vi "WILT.vi"() -> ()   [LabVIEW 2016] (continued)
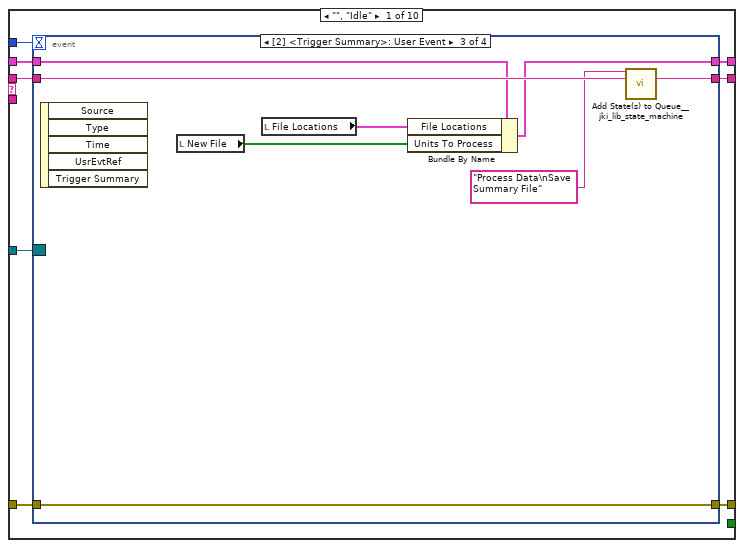
[diagram p2: hidden frame]
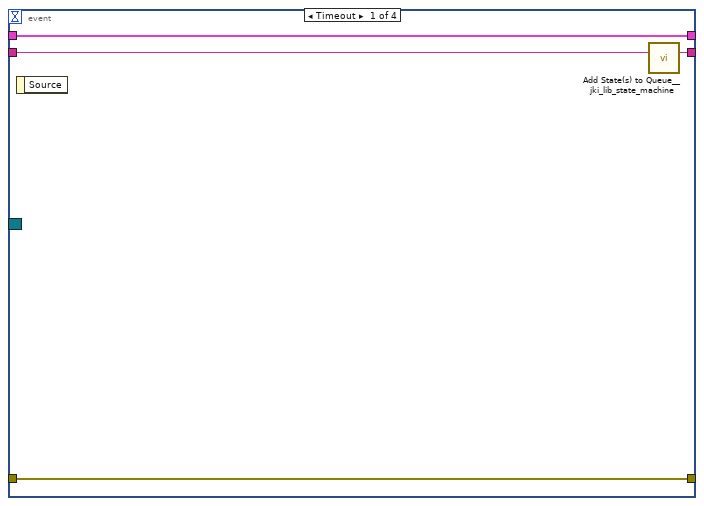
[diagram p3: hidden frame]
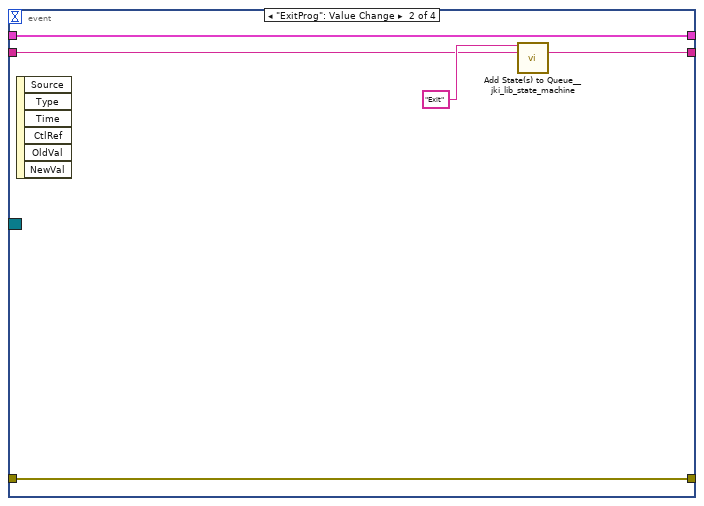
[diagram p4: hidden frame]
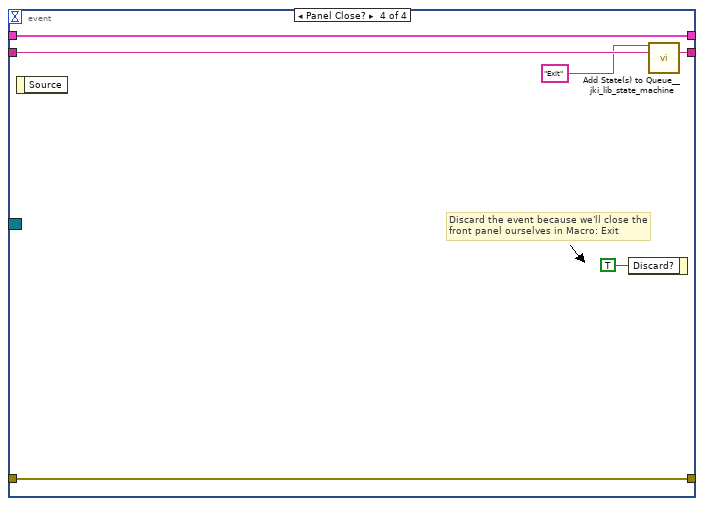
[diagram p5: hidden frame]
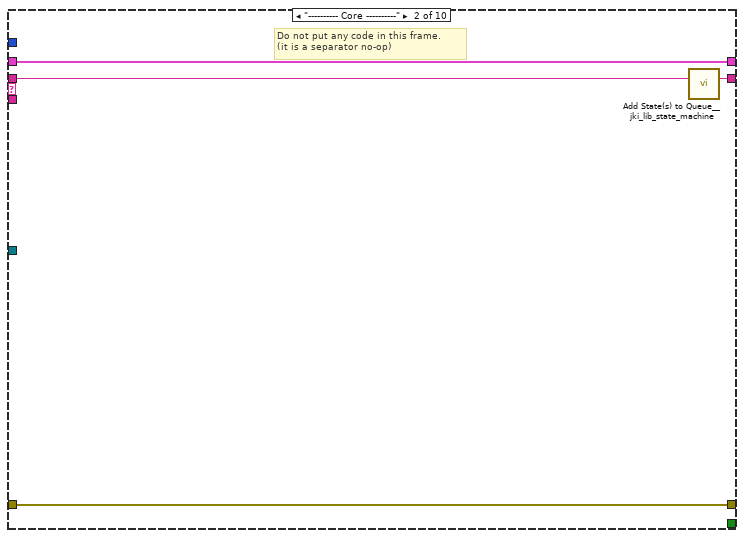
[diagram p6: hidden frame]
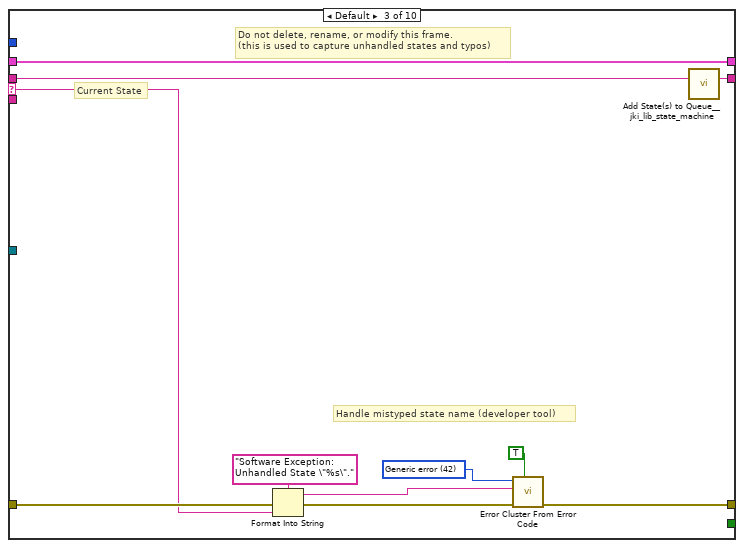
[diagram p7: hidden frame]
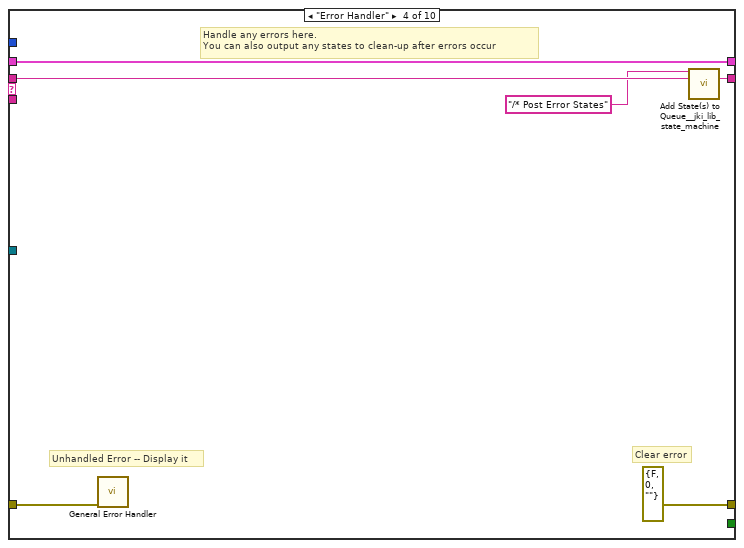
[diagram p8: hidden frame]
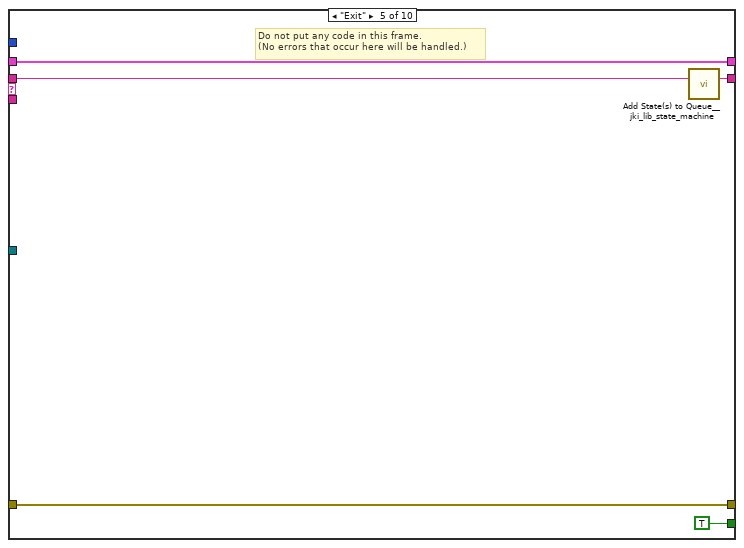
[diagram p9: hidden frame]
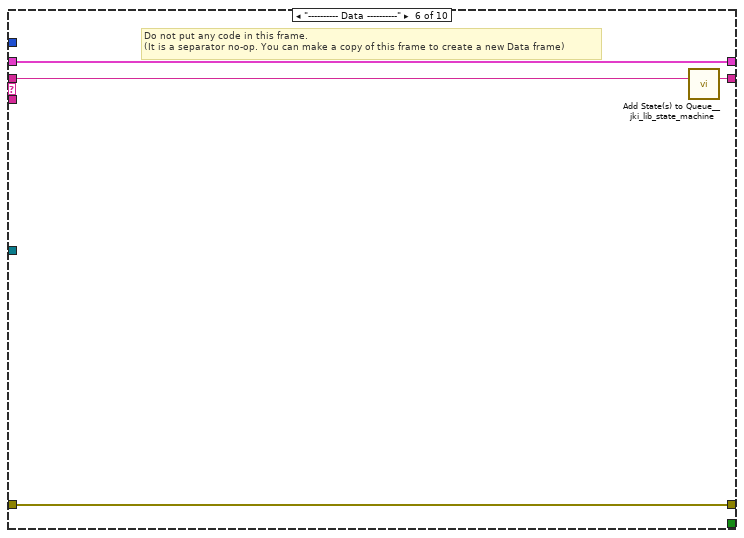
[diagram p10: hidden frame]
        n2035 = call <vilib>:"Add State(s) to Queue__jki_lib_state_machine.vi"("State(s) in (\"\")"=w4584) -> ("States Out"=w4583:string)  [unwired: 14 in]
      }
      frame "Update Filenames" {
        # "This takes alot of time to do...i cannot have 1 sec scan rate\nat this time...I set to 10 sec"
        n2036 = Unbundle By Name(w4604) -> ("First Time Through?"=w4601:bool[], "File Refnums"=w4587:refnum<file>[])
        n2037 = local read "Station Test State Cluster 2"() -> (w4586:T7)
        n2038 = local read "File Locations"() -> (w4602:T17[])
        n2039 = Wait on Notification(notifier=w4592, error in (no error)=w4591) -> (notification=w4589:T3[], error out=w4590:errorcluster)  [unwired: 2 in, 2 out]
        n2040 = call "WILT Save File.vi"("File Locations"=w4602, "Station Test State Cluster 2"=w4586, "Array in"=w4589, "File References In"=w4587, "Fisrt Time Through?"=w4601, "Error In"=w4590) -> ("File Locations Out"=w4600:T17[], "First Time Through Out"=w4585:bool[], "File References Out"=w4588:refnum<file>[], "New File"=w4599:bool[], "Error Out"=w4595:errorcluster)  [unwired: 5 in]
        "New File" <- w4599
        n2041 = Or Array Elements(Boolean array=w4599) -> (logical OR=w4598:bool)
        n2042 = case shown="True" w4598 {
          tunnel: w4597 -> [w4609 w4614]
          tunnel: [w4609 w4613] -> w4596
          tunnel: w4595 -> [w4608 w4612]
          tunnel: [w4608 w4611] -> w4594
          tunnel: ["" "Prepare for Save"] -> w4593
          frame False {
          }
          frame True {
            n2043 = Generate User Event(user event=w4614, event data cluster=TRUE ("Trigger"), error in=w4612) -> (user event out=w4613:refnum<user-event>, error out=w4611:errorcluster)  [unwired: 1 in]
          }
        }
        n2044 = Bundle By Name(cluster=w4604, "File Locations"=w4600, "First Time Through?"=w4585, "File Refnums"=w4588) -> (w4603:T36)
        n2045 = call <vilib>:"Add State(s) to Queue__jki_lib_state_machine.vi"("State(s) in Front (\"\")"=w4593, "State(s) in (\"\")"=w4606) -> ("States Out"=w4605:string)  [unwired: 13 in]
      }
    }
    n2046 = local read "Debug 2"() -> (w4468:bool)
    n2047 = case shown="False" w4468 {
      tunnel: w4471 -> [_ w4486]
      tunnel: [w4481 w4483] -> w4469
      tunnel: w4470 -> [w4481 w4485]
      frame False {
      }
      frame True {
        n2048 = Build Array (concatenate)(w4485, w4486) -> (w4482:string[])
        "Test State array 4" <- w4482
        n2049 = Array Size(array=w4482) -> (size(s)=w4484:i32)
        n2050 = case shown="100" w4484 {
          tunnel: [w4487 w4490] -> w4483
          tunnel: w4482 -> [w4487 w4491]
          frame 0, Default {
          }
          frame 100 {
            n2051 = Delete From Array(array=w4491, length=5, index=0) -> (array with subset deleted=w4490:string[])  [unwired: 1 out]
          }
        }
      }
    }
  }
  n2052 = while "Summary File Processing" {
    shift-right: [w4620] -> _
    shift-left: _ -> [w4619]
    shift-right: [w4623] -> _
    shift-left: _ -> [w4617]
    shift-right: [w4622] -> _
    shift-left: w48 -> [w4624]
    tunnel: w43 -> [w4616]
    stop <- w4621 stop-if-true
    w4618 = -1  # Timeout
    # "Summary File Processing"
    n2053 = call <vilib>:"Parse State Queue__jki_lib_state_machine.vi"("State Queue"=w4624, "Error In (no error)"=w4617) -> ("Remaining States"=w4626:string, "Current State"=w4627:string, "Arguments"=w4625:string)  [unwired: 11 in]
    n2054 = case shown="\"Process Data\"" w4627 {
      selector: w4627 -> [_ _ w4663 _ _ _ _ _ _ _]
      tunnel: w4626 -> [w4635 w4662 w4667 w4679 w4684 w4688 w4695 w4704 w4715 w4723]
      tunnel: w4625 -> [_ _ _ _ _ _ _ _ _ _]
      tunnel: w4619 -> [w4633 w4659 w4665 w4676 w4682 w4685 _ w4701 w4710 w4721]
      tunnel: [w4632 w4660 w4669 errorcluster {"status"=FALSE, "code"=0, "source"=""} ("error out") w4681 w4686 w4692 w4702 w4713 w4716] -> w4623
      tunnel: w4617 -> [w4631 w4660 w4668 w4675 w4681 w4686 w4692 w4702 w4713 w4717]
      tunnel: [w4634 w4661 w4666 w4678 w4683 w4687 w4694 w4703 w4714 w4722] -> w4622
      tunnel: [_ _ _ _ TRUE _ _ _ _ _] -> w4621
      tunnel: [w4630 w4659 w4665 w4676 w4682 w4685 w4693 w4701 w4709 w4721] -> w4620
      tunnel: w4618 -> [w4629 _ _ _ _ _ _ _ _ _]
      tunnel: w4616 -> [w4628 _ _ _ _ _ _ _ _ _]
      frame "", "Idle" {
        n2055 = event shown="[2] <Trigger Summary>: User Event" {
          selector: w4628 -> [_ _ _ _]
          dyn-events: _ -> [_ _ _ _]
          timeout: w4629 -> [_ _ _ _]
          tunnel: w4635 -> [w4639 w4641 w4651 w4658]
          tunnel: [w4638 w4642 w4652 w4657] -> w4634
          tunnel: w4633 -> [w4636 w4644 w4650 w4655]
          tunnel: [w4637 w4640 w4645 w4656] -> w4632
          tunnel: w4631 -> [w4637 w4640 w4645 w4656]
          tunnel: [w4636 w4644 w4649 w4655] -> w4630
          event Timeout {
            n2056 = event-data() -> ()  [unwired: 1 in, 1 out]
            n2057 = call <vilib>:"Add State(s) to Queue__jki_lib_state_machine.vi"("State(s) in (\"\")"=w4639) -> ("States Out"=w4638:string)  [unwired: 14 in]
          }
          event "ExitProg": Value Change {
            n2058 = event-data() -> ()  [unwired: 1 in, 6 out]
            n2059 = call <vilib>:"Add State(s) to Queue__jki_lib_state_machine.vi"("State(s) in Front (\"\")"="Exit" ("State(s) in Front (\"\")"), "State(s) in (\"\")"=w4641) -> ("States Out"=w4642:string)  [unwired: 13 in]
          }
          event User Event {
            n2060 = event-data() -> ()  [unwired: 1 in, 5 out]
            n2061 = local read "New File"() -> (w4648:bool[])
            n2062 = local read "File Locations"() -> (w4646:T17[])
            n2063 = Bundle By Name(cluster=w4650, "File Locations"=w4646, "Units To Process"=w4648) -> (w4649:T37)
            n2064 = call <vilib>:"Add State(s) to Queue__jki_lib_state_machine.vi"("State(s) in Front (\"\")"="Process Data\nSave Summary File" ("State(s) in Front (\"\")"), "State(s) in (\"\")"=w4651) -> ("States Out"=w4652:string)  [unwired: 13 in]
          }
          event Panel Close? {
            # "Discard the event because we'll close the front panel ourselves in Macro: Exit"
            n2065 = event-data() -> ()  [unwired: 1 in, 1 out]
            n2066 = event-data("Discard?"=TRUE) -> ()  [unwired: 1 in, 1 out]
            n2067 = call <vilib>:"Add State(s) to Queue__jki_lib_state_machine.vi"("State(s) in Front (\"\")"="Exit", "State(s) in (\"\")"=w4658) -> ("States Out"=w4657:string)  [unwired: 13 in]
          }
        }
      }
      frame "---------- Core ----------" {
        # "Do not put any code in this frame.\n(it is a separator no-op)"
        n2068 = call <vilib>:"Add State(s) to Queue__jki_lib_state_machine.vi"("State(s) in (\"\")"=w4662) -> ("States Out"=w4661:string)  [unwired: 14 in]
      }
      frame Default {
        w4672 = 42 items=["No error", "Argument error", "Memory is full", "Out of zone", "End of file", "File already open", "Generic file I/O error", "File not found", "File permission error", "Disk is full", "Duplicate path", "Too many files open", "System feature not enabled", "Resource file not found", "Cannot add resource", "Resource not found", "Image not found", "Image memory error", "Pen does not exist", "Config type invalid", "Config token not found", "Config parse error", "Config memory error", "Bad external code format", "Bad external code offset", "External code not present", "Null window", "Destroy window error", "Null menu", "Print aborted", "Bad print record", "Print driver error", "Windows error during printing", "Memory error during printing", "Print dialog error", "Generic print error", "Invalid device refnum", "Device not found", "Device parameter error", "Device unit error", "Cannot open device", "Device call aborted", "Generic error", "Cancelled by user", "Object ID too low", "Object ID too high", "Object not in heap", "Unknown heap", "Unknown object (invalid DefProc)", "Unknown object (DefProc not in table)", "Message out of range", "Invalid (null) method", "Unknown message", "Manager call not supported", "Bad address", "Network operation in progress", "Network operation timed out", "Connection is busy", "Network attribute not supported", "Network error", "Address in use", "System out of memory", "Connection aborted", "Connection refused", "Not connected", "Already connected", "Connection closed", "Initialization error (interapplication manager)", "Bad occurrence", "Wait on unbound occurrence handler", "Occurrence queue overflow", "Datalog type conflict", "Unused", "Unrecognized type (interapplication manager)", "Memory corrupt", "Failed to make temporary DLL", "Old CIN version", "Drag socket not found", "Failed to load drop-object", "Failed to register OLE object", "Failed to release OLE object", "Format specifier type mismatch", "Unknown format specifier", "Too few format specifiers", "Too many format specifiers", "Scan failed", "Newer CIN version", "Error converting to variant", "Runtime menu error", "Password tampered", "Variant attribute not found", "Incompatible variant data type", "Event data is not available", "Event Store is not present", "Occurrence is not found", "Event Queue is not created", "Event info is not available", "Refnum passed is NULL", "Error retrieving Class GUID", "Error retrieving CoClass GUID", "Error retrieving TypeLib GUID.", "Bad built application magic bytes.", "Specific driver is different from the specific driver associated with the Logical Name.", "There is no session opened to the class driver.", "Max Error", "MAX - Error with config objects", "MAX - Error loading configuration", "MAX - Group not supported"]
        # "Current State"
        # "Do not delete, rename, or modify this frame.\n(this is used to capture unhandled states and typos)"
        # "Handle mistyped state name (developer tool)"
        n2069 = Format Into String(format string="Software Exception: Unhandled State \"%s\"." ("message"), error in=w4668, w4663) -> (resulting string=w4671:string, error out=w4670:errorcluster)  [unwired: 1 in]
        n2070 = call <vilib>:"Error Cluster From Error Code.vi"("show call chain? (False)"=TRUE, "error in (no error)"=w4670, "error message (\"\")"=w4671, "error code (0)"=w4672) -> ("error out"=w4669:errorcluster)  [unwired: 5 in]
        n2071 = call <vilib>:"Add State(s) to Queue__jki_lib_state_machine.vi"("State(s) in (\"\")"=w4667) -> ("States Out"=w4666:string)  [unwired: 14 in]
      }
      frame "Error Handler" {
        # "Unhandled Error -- Display it"
        # "Handle any errors here.\nYou can also output any states to clean-up after errors occur"
        # "Clear error"
        n2072 = call <vilib>:"General Error Handler.vi"("error in (no error)"=w4675) -> ()  [unwired: 10 in, 5 out]
        n2073 = call <vilib>:"Add State(s) to Queue__jki_lib_state_machine.vi"("State(s) in Front (\"\")"="/* Post Error States", "State(s) in (\"\")"=w4679) -> ("States Out"=w4678:string)  [unwired: 13 in]
      }
      frame "Exit" {
        # "Do not put any code in this frame.\n(No errors that occur here will be handled.)"
        n2074 = call <vilib>:"Add State(s) to Queue__jki_lib_state_machine.vi"("State(s) in (\"\")"=w4684) -> ("States Out"=w4683:string)  [unwired: 14 in]
      }
      frame "---------- Data ----------" {
        # "Do not put any code in this frame.\n(It is a separator no-op. You can make a copy of this frame to create a new Data frame)"
        n2075 = call <vilib>:"Add State(s) to Queue__jki_lib_state_machine.vi"("State(s) in (\"\")"=w4688) -> ("States Out"=w4687:string)  [unwired: 14 in]
      }
      frame "Data: Initialize" {
        n2076 = while {
          tunnel: [w4698] -> w4691
          tunnel: [w4696] -> w4690
          tunnel: [w4697] -> w4689
          stop <- w4700 stop-if-true
          w4696 = T9[] [{"Cycle Time (Minutes)"=0.0, "L1 Current (Amps)"=0.0, "L2 Current (Amps)"=0.0, "TC Temperature (Deg F)"=0.0, "Voltage (Volts)"=0.0, "Voltage-208 (Volts)"=0.0, "208V Switch (Ohms)"=0.0, "Cycle Number"=0}, {"Cycle Time (Minutes)"=0.0, "L1 Current (Amps)"=0.0, "L2 Current (Amps)"=0.0, "TC Temperature (Deg F)"=0.0, "Voltage (Volts)"=0.0, "Voltage-208 (Volts)"=0.0, "208V Switch (Ohms)"=0.0, "Cycle Number"=0}, {"Cycle Time (Minutes)"=0.0, "L1 Current (Amps)"=0.0, "L2 Current (Amps)"=0.0, "TC Temperature (Deg F)"=0.0, "Voltage (Volts)"=0.0, "Voltage-208 (Volts)"=0.0, "208V Switch (Ohms)"=0.0, "Cycle Number"=0}, {"Cycle Time (Minutes)"=0.0, "L1 Current (Amps)"=0.0, "L2 Current (Amps)"=0.0, "TC Temperature (Deg F)"=0.0, "Voltage (Volts)"=0.0, "Voltage-208 (Volts)"=0.0, "208V Switch (Ohms)"=0.0, "Cycle Number"=0}, {"Cycle Time (Minutes)"=0.0, "L1 Current (Amps)"=0.0, "L2 Current (Amps)"=0.0, "TC Temperature (Deg F)"=0.0, "Voltage (Volts)"=0.0, "Voltage-208 (Volts)"=0.0, "208V Switch (Ohms)"=0.0, "Cycle Number"=0}, {"Cycle Time (Minutes)"=0.0, "L1 Current (Amps)"=0.0, "L2 Current (Amps)"=0.0, "TC Temperature (Deg F)"=0.0, "Voltage (Volts)"=0.0, "Voltage-208 (Volts)"=0.0, "208V Switch (Ohms)"=0.0, "Cycle Number"=0}, {"Cycle Time (Minutes)"=0.0, "L1 Current (Amps)"=0.0, "L2 Current (Amps)"=0.0, "TC Temperature (Deg F)"=0.0, "Voltage (Volts)"=0.0, "Voltage-208 (Volts)"=0.0, "208V Switch (Ohms)"=0.0, "Cycle Number"=0}, {"Cycle Time (Minutes)"=0.0, "L1 Current (Amps)"=0.0, "L2 Current (Amps)"=0.0, "TC Temperature (Deg F)"=0.0, "Voltage (Volts)"=0.0, "Voltage-208 (Volts)"=0.0, "208V Switch (Ohms)"=0.0, "Cycle Number"=0}, {"Cycle Time (Minutes)"=0.0, "L1 Current (Amps)"=0.0, "L2 Current (Amps)"=0.0, "TC Temperature (Deg F)"=0.0, "Voltage (Volts)"=0.0, "Voltage-208 (Volts)"=0.0, "208V Switch (Ohms)"=0.0, "Cycle Number"=0}, {"Cycle Time (Minutes)"=0.0, "L1 Current (Amps)"=0.0, "L2 Current (Amps)"=0.0, "TC Temperature (Deg F)"=0.0, "Voltage (Volts)"=0.0, "Voltage-208 (Volts)"=0.0, "208V Switch (Ohms)"=0.0, "Cycle Number"=0}, {"Cycle Time (Minutes)"=0.0, "L1 Current (Amps)"=0.0, "L2 Current (Amps)"=0.0, "TC Temperature (Deg F)"=0.0, "Voltage (Volts)"=0.0, "Voltage-208 (Volts)"=0.0, "208V Switch (Ohms)"=0.0, "Cycle Number"=0}, {"Cycle Time (Minutes)"=0.0, "L1 Current (Amps)"=0.0, "L2 Current (Amps)"=0.0, "TC Temperature (Deg F)"=0.0, "Voltage (Volts)"=0.0, "Voltage-208 (Volts)"=0.0, "208V Switch (Ohms)"=0.0, "Cycle Number"=0}, {"Cycle Time (Minutes)"=0.0, "L1 Current (Amps)"=0.0, "L2 Current (Amps)"=0.0, "TC Temperature (Deg F)"=0.0, "Voltage (Volts)"=0.0, "Voltage-208 (Volts)"=0.0, "208V Switch (Ohms)"=0.0, "Cycle Number"=0}, {"Cycle Time (Minutes)"=0.0, "L1 Current (Amps)"=0.0, "L2 Current (Amps)"=0.0, "TC Temperature (Deg F)"=0.0, "Voltage (Volts)"=0.0, "Voltage-208 (Volts)"=0.0, "208V Switch (Ohms)"=0.0, "Cycle Number"=0}, {"Cycle Time (Minutes)"=0.0, "L1 Current (Amps)"=0.0, "L2 Current (Amps)"=0.0, "TC Temperature (Deg F)"=0.0, "Voltage (Volts)"=0.0, "Voltage-208 (Volts)"=0.0, "208V Switch (Ohms)"=0.0, "Cycle Number"=0}, {"Cycle Time (Minutes)"=0.0, "L1 Current (Amps)"=0.0, "L2 Current (Amps)"=0.0, "TC Temperature (Deg F)"=0.0, "Voltage (Volts)"=0.0, "Voltage-208 (Volts)"=0.0, "208V Switch (Ohms)"=0.0, "Cycle Number"=0}, {"Cycle Time (Minutes)"=0.0, "L1 Current (Amps)"=0.0, "L2 Current (Amps)"=0.0, "TC Temperature (Deg F)"=0.0, "Voltage (Volts)"=0.0, "Voltage-208 (Volts)"=0.0, "208V Switch (Ohms)"=0.0, "Cycle Number"=0}, {"Cycle Time (Minutes)"=0.0, "L1 Current (Amps)"=0.0, "L2 Current (Amps)"=0.0, "TC Temperature (Deg F)"=0.0, "Voltage (Volts)"=0.0, "Voltage-208 (Volts)"=0.0, "208V Switch (Ohms)"=0.0, "Cycle Number"=0}, {"Cycle Time (Minutes)"=0.0, "L1 Current (Amps)"=0.0, "L2 Current (Amps)"=0.0, "TC Temperature (Deg F)"=0.0, "Voltage (Volts)"=0.0, "Voltage-208 (Volts)"=0.0, "208V Switch (Ohms)"=0.0, "Cycle Number"=0}, {"Cycle Time (Minutes)"=0.0, "L1 Current (Amps)"=0.0, "L2 Current (Amps)"=0.0, "TC Temperature (Deg F)"=0.0, "Voltage (Volts)"=0.0, "Voltage-208 (Volts)"=0.0, "208V Switch (Ohms)"=0.0, "Cycle Number"=0}, {"Cycle Time (Minutes)"=0.0, "L1 Current (Amps)"=0.0, "L2 Current (Amps)"=0.0, "TC Temperature (Deg F)"=0.0, "Voltage (Volts)"=0.0, "Voltage-208 (Volts)"=0.0, "208V Switch (Ohms)"=0.0, "Cycle Number"=0}, {"Cycle Time (Minutes)"=0.0, "L1 Current (Amps)"=0.0, "L2 Current (Amps)"=0.0, "TC Temperature (Deg F)"=0.0, "Voltage (Volts)"=0.0, "Voltage-208 (Volts)"=0.0, "208V Switch (Ohms)"=0.0, "Cycle Number"=0}, {"Cycle Time (Minutes)"=0.0, "L1 Current (Amps)"=0.0, "L2 Current (Amps)"=0.0, "TC Temperature (Deg F)"=0.0, "Voltage (Volts)"=0.0, "Voltage-208 (Volts)"=0.0, "208V Switch (Ohms)"=0.0, "Cycle Number"=0}, {"Cycle Time (Minutes)"=0.0, "L1 Current (Amps)"=0.0, "L2 Current (Amps)"=0.0, "TC Temperature (Deg F)"=0.0, "Voltage (Volts)"=0.0, "Voltage-208 (Volts)"=0.0, "208V Switch (Ohms)"=0.0, "Cycle Number"=0}, {"Cycle Time (Minutes)"=0.0, "L1 Current (Amps)"=0.0, "L2 Current (Amps)"=0.0, "TC Temperature (Deg F)"=0.0, "Voltage (Volts)"=0.0, "Voltage-208 (Volts)"=0.0, "208V Switch (Ohms)"=0.0, "Cycle Number"=0}, {"Cycle Time (Minutes)"=0.0, "L1 Current (Amps)"=0.0, "L2 Current (Amps)"=0.0, "TC Temperature (Deg F)"=0.0, "Voltage (Volts)"=0.0, "Voltage-208 (Volts)"=0.0, "208V Switch (Ohms)"=0.0, "Cycle Number"=0}, {"Cycle Time (Minutes)"=0.0, "L1 Current (Amps)"=0.0, "L2 Current (Amps)"=0.0, "TC Temperature (Deg F)"=0.0, "Voltage (Volts)"=0.0, "Voltage-208 (Volts)"=0.0, "208V Switch (Ohms)"=0.0, "Cycle Number"=0}, {"Cycle Time (Minutes)"=0.0, "L1 Current (Amps)"=0.0, "L2 Current (Amps)"=0.0, "TC Temperature (Deg F)"=0.0, "Voltage (Volts)"=0.0, "Voltage-208 (Volts)"=0.0, "208V Switch (Ohms)"=0.0, "Cycle Number"=0}, {"Cycle Time (Minutes)"=0.0, "L1 Current (Amps)"=0.0, "L2 Current (Amps)"=0.0, "TC Temperature (Deg F)"=0.0, "Voltage (Volts)"=0.0, "Voltage-208 (Volts)"=0.0, "208V Switch (Ohms)"=0.0, "Cycle Number"=0}, {"Cycle Time (Minutes)"=0.0, "L1 Current (Amps)"=0.0, "L2 Current (Amps)"=0.0, "TC Temperature (Deg F)"=0.0, "Voltage (Volts)"=0.0, "Voltage-208 (Volts)"=0.0, "208V Switch (Ohms)"=0.0, "Cycle Number"=0}, {"Cycle Time (Minutes)"=0.0, "L1 Current (Amps)"=0.0, "L2 Current (Amps)"=0.0, "TC Temperature (Deg F)"=0.0, "Voltage (Volts)"=0.0, "Voltage-208 (Volts)"=0.0, "208V Switch (Ohms)"=0.0, "Cycle Number"=0}, {"Cycle Time (Minutes)"=0.0, "L1 Current (Amps)"=0.0, "L2 Current (Amps)"=0.0, "TC Temperature (Deg F)"=0.0, "Voltage (Volts)"=0.0, "Voltage-208 (Volts)"=0.0, "208V Switch (Ohms)"=0.0, "Cycle Number"=0}, {"Cycle Time (Minutes)"=0.0, "L1 Current (Amps)"=0.0, "L2 Current (Amps)"=0.0, "TC Temperature (Deg F)"=0.0, "Voltage (Volts)"=0.0, "Voltage-208 (Volts)"=0.0, "208V Switch (Ohms)"=0.0, "Cycle Number"=0}, {"Cycle Time (Minutes)"=0.0, "L1 Current (Amps)"=0.0, "L2 Current (Amps)"=0.0, "TC Temperature (Deg F)"=0.0, "Voltage (Volts)"=0.0, "Voltage-208 (Volts)"=0.0, "208V Switch (Ohms)"=0.0, "Cycle Number"=0}, {"Cycle Time (Minutes)"=0.0, "L1 Current (Amps)"=0.0, "L2 Current (Amps)"=0.0, "TC Temperature (Deg F)"=0.0, "Voltage (Volts)"=0.0, "Voltage-208 (Volts)"=0.0, "208V Switch (Ohms)"=0.0, "Cycle Number"=0}, {"Cycle Time (Minutes)"=0.0, "L1 Current (Amps)"=0.0, "L2 Current (Amps)"=0.0, "TC Temperature (Deg F)"=0.0, "Voltage (Volts)"=0.0, "Voltage-208 (Volts)"=0.0, "208V Switch (Ohms)"=0.0, "Cycle Number"=0}, {"Cycle Time (Minutes)"=0.0, "L1 Current (Amps)"=0.0, "L2 Current (Amps)"=0.0, "TC Temperature (Deg F)"=0.0, "Voltage (Volts)"=0.0, "Voltage-208 (Volts)"=0.0, "208V Switch (Ohms)"=0.0, "Cycle Number"=0}, {"Cycle Time (Minutes)"=0.0, "L1 Current (Amps)"=0.0, "L2 Current (Amps)"=0.0, "TC Temperature (Deg F)"=0.0, "Voltage (Volts)"=0.0, "Voltage-208 (Volts)"=0.0, "208V Switch (Ohms)"=0.0, "Cycle Number"=0}, {"Cycle Time (Minutes)"=0.0, "L1 Current (Amps)"=0.0, "L2 Current (Amps)"=0.0, "TC Temperature (Deg F)"=0.0, "Voltage (Volts)"=0.0, "Voltage-208 (Volts)"=0.0, "208V Switch (Ohms)"=0.0, "Cycle Number"=0}, {"Cycle Time (Minutes)"=0.0, "L1 Current (Amps)"=0.0, "L2 Current (Amps)"=0.0, "TC Temperature (Deg F)"=0.0, "Voltage (Volts)"=0.0, "Voltage-208 (Volts)"=0.0, "208V Switch (Ohms)"=0.0, "Cycle Number"=0}, {"Cycle Time (Minutes)"=0.0, "L1 Current (Amps)"=0.0, "L2 Current (Amps)"=0.0, "TC Temperature (Deg F)"=0.0, "Voltage (Volts)"=0.0, "Voltage-208 (Volts)"=0.0, "208V Switch (Ohms)"=0.0, "Cycle Number"=0}, {"Cycle Time (Minutes)"=0.0, "L1 Current (Amps)"=0.0, "L2 Current (Amps)"=0.0, "TC Temperature (Deg F)"=0.0, "Voltage (Volts)"=0.0, "Voltage-208 (Volts)"=0.0, "208V Switch (Ohms)"=0.0, "Cycle Number"=0}, {"Cycle Time (Minutes)"=0.0, "L1 Current (Amps)"=0.0, "L2 Current (Amps)"=0.0, "TC Temperature (Deg F)"=0.0, "Voltage (Volts)"=0.0, "Voltage-208 (Volts)"=0.0, "208V Switch (Ohms)"=0.0, "Cycle Number"=0}, {"Cycle Time (Minutes)"=0.0, "L1 Current (Amps)"=0.0, "L2 Current (Amps)"=0.0, "TC Temperature (Deg F)"=0.0, "Voltage (Volts)"=0.0, "Voltage-208 (Volts)"=0.0, "208V Switch (Ohms)"=0.0, "Cycle Number"=0}, {"Cycle Time (Minutes)"=0.0, "L1 Current (Amps)"=0.0, "L2 Current (Amps)"=0.0, "TC Temperature (Deg F)"=0.0, "Voltage (Volts)"=0.0, "Voltage-208 (Volts)"=0.0, "208V Switch (Ohms)"=0.0, "Cycle Number"=0}, {"Cycle Time (Minutes)"=0.0, "L1 Current (Amps)"=0.0, "L2 Current (Amps)"=0.0, "TC Temperature (Deg F)"=0.0, "Voltage (Volts)"=0.0, "Voltage-208 (Volts)"=0.0, "208V Switch (Ohms)"=0.0, "Cycle Number"=0}, {"Cycle Time (Minutes)"=0.0, "L1 Current (Amps)"=0.0, "L2 Current (Amps)"=0.0, "TC Temperature (Deg F)"=0.0, "Voltage (Volts)"=0.0, "Voltage-208 (Volts)"=0.0, "208V Switch (Ohms)"=0.0, "Cycle Number"=0}, {"Cycle Time (Minutes)"=0.0, "L1 Current (Amps)"=0.0, "L2 Current (Amps)"=0.0, "TC Temperature (Deg F)"=0.0, "Voltage (Volts)"=0.0, "Voltage-208 (Volts)"=0.0, "208V Switch (Ohms)"=0.0, "Cycle Number"=0}, {"Cycle Time (Minutes)"=0.0, "L1 Current (Amps)"=0.0, "L2 Current (Amps)"=0.0, "TC Temperature (Deg F)"=0.0, "Voltage (Volts)"=0.0, "Voltage-208 (Volts)"=0.0, "208V Switch (Ohms)"=0.0, "Cycle Number"=0}, {"Cycle Time (Minutes)"=0.0, "L1 Current (Amps)"=0.0, "L2 Current (Amps)"=0.0, "TC Temperature (Deg F)"=0.0, "Voltage (Volts)"=0.0, "Voltage-208 (Volts)"=0.0, "208V Switch (Ohms)"=0.0, "Cycle Number"=0}, {"Cycle Time (Minutes)"=0.0, "L1 Current (Amps)"=0.0, "L2 Current (Amps)"=0.0, "TC Temperature (Deg F)"=0.0, "Voltage (Volts)"=0.0, "Voltage-208 (Volts)"=0.0, "208V Switch (Ohms)"=0.0, "Cycle Number"=0}, {"Cycle Time (Minutes)"=0.0, "L1 Current (Amps)"=0.0, "L2 Current (Amps)"=0.0, "TC Temperature (Deg F)"=0.0, "Voltage (Volts)"=0.0, "Voltage-208 (Volts)"=0.0, "208V Switch (Ohms)"=0.0, "Cycle Number"=0}, {"Cycle Time (Minutes)"=0.0, "L1 Current (Amps)"=0.0, "L2 Current (Amps)"=0.0, "TC Temperature (Deg F)"=0.0, "Voltage (Volts)"=0.0, "Voltage-208 (Volts)"=0.0, "208V Switch (Ohms)"=0.0, "Cycle Number"=0}, {"Cycle Time (Minutes)"=0.0, "L1 Current (Amps)"=0.0, "L2 Current (Amps)"=0.0, "TC Temperature (Deg F)"=0.0, "Voltage (Volts)"=0.0, "Voltage-208 (Volts)"=0.0, "208V Switch (Ohms)"=0.0, "Cycle Number"=0}, {"Cycle Time (Minutes)"=0.0, "L1 Current (Amps)"=0.0, "L2 Current (Amps)"=0.0, "TC Temperature (Deg F)"=0.0, "Voltage (Volts)"=0.0, "Voltage-208 (Volts)"=0.0, "208V Switch (Ohms)"=0.0, "Cycle Number"=0}, {"Cycle Time (Minutes)"=0.0, "L1 Current (Amps)"=0.0, "L2 Current (Amps)"=0.0, "TC Temperature (Deg F)"=0.0, "Voltage (Volts)"=0.0, "Voltage-208 (Volts)"=0.0, "208V Switch (Ohms)"=0.0, "Cycle Number"=0}]  # WILT Summary Array
          w4697 = bool[] [FALSE, FALSE, FALSE, FALSE, FALSE, FALSE, FALSE, FALSE, FALSE, FALSE, FALSE, FALSE, FALSE, FALSE, FALSE, FALSE, FALSE, FALSE, FALSE, FALSE, FALSE, FALSE, FALSE, FALSE, FALSE, FALSE, FALSE, FALSE, FALSE, FALSE, FALSE, FALSE, FALSE, FALSE, FALSE, FALSE, FALSE, FALSE, FALSE, FALSE, FALSE, FALSE, FALSE, FALSE, FALSE, FALSE, FALSE, FALSE, FALSE, FALSE, FALSE, FALSE, FALSE, FALSE, FALSE, FALSE]  # Units To Process
          n2077 = local read "Initialization Complete"() -> (w4700:bool)
          n2078 = local read "File Locations"() -> (w4698:T17[])
          n2079 = Wait Until Next ms Multiple(millisecond multiple=u32 100) -> ()  [unwired: 1 out]
        }
        n2080 = Bundle("File Locations"=w4691, "WILT Summary Array"=w4690, "Units To Process"=w4689) -> (w4693:T37)  [unwired: 1 in]
        n2081 = call <vilib>:"Add State(s) to Queue__jki_lib_state_machine.vi"("State(s) in (\"\")"=w4695) -> ("States Out"=w4694:string)  [unwired: 14 in]
      }
      frame "---------- Summary File Process ----------" {
        n2082 = call <vilib>:"Add State(s) to Queue__jki_lib_state_machine.vi"("State(s) in (\"\")"=w4704) -> ("States Out"=w4703:string)  [unwired: 14 in]
      }
      frame "Process Data" {
        # "Loops through all files and computes\ncomplete files. Including Cycle Time"
        n2083 = Unbundle By Name(w4710) -> ("WILT Summary Array"=w4706:T9[], "Units To Process"=w4708:bool[], "File Locations"=w4712:T17[])
        n2084 = call "WILT Process Cycle Data.vi"("WILT Summary Input"=w4706, "Inverter File Headers"=string[] ["Date", "Time (24 Hour Format)", "Cycle Time (Minutes)", "L1 Current (Amps)", "L2 Current (Amps)", "TC Temperature (Deg F)", "Voltage (Volts)", "Voltage-208 (Volts)", "208V Switch (Ohms)", "Cycle Number"], "File Locations"=w4712, "New File"=w4708) -> ("Units to Process"=w4707:bool[], "WILT Summary Output"=w4705:T9[])  [unwired: 6 in]
        "Previous Run Statistics" <- w4705
        n2085 = Bundle By Name(cluster=w4710, "WILT Summary Array"=w4705, "Units To Process"=w4707) -> (w4709:T37)
        n2086 = call <vilib>:"Add State(s) to Queue__jki_lib_state_machine.vi"("State(s) in (\"\")"=w4715) -> ("States Out"=w4714:string)  [unwired: 14 in]
      }
      frame "Save Summary File" {
        # "This could consume memory\nkeep a watch"
        # "Loops through files and saves data\nto summary file by cycle number"
        n2087 = Unbundle By Name(w4721) -> ("Units To Process"=w4720:bool[], "File Locations"=w4719:T17[], "WILT Summary Array"=w4718:T9[])
        n2088 = for {
          tunnel: w4720 -> [w4728] mode=indexing
          tunnel: w4719 -> [w4727] mode=indexing
          tunnel: w4718 -> [w4726] mode=indexing
          shift-right: [w4724] -> w4716
          shift-left: w4717 -> [w4725]
          n2089 = case shown="True" w4728 {
            tunnel: w4727 -> [_ w4738]
            tunnel: w4726 -> [_ w4733]
            tunnel: w4725 -> [w4729 w4732]
            tunnel: [w4729 w4732] -> w4724
            frame False {
            }
            frame True {
              n2090 = Unbundle By Name(w4738) -> ("Data File Paths.Summary"=w4737:path)
              n2091 = call "WILT Format Summary File.vi"("WILT Summary Cluster Input"=w4733) -> ("Summary Data"=w4730:string[])  [unwired: 10 in]
              n2092 = call "Save File Check and Fix Summary File.vi"("LV Program"=Save_File_DOE_LabView_Program."Dryer", "file path (dialog if empty)"=w4737) -> ("Summary Path"=w4734:path)  [unwired: 8 in, 1 out]
              n2093 = call-poly <vilib>:"Write Delimited Spreadsheet.vi"("file path (dialog if empty)"=w4734, "1D data"=w4730, "append to file? (new file:F)"=TRUE, "delimiter (\\t)"="," ("delimiter (\\t)")) -> ()  [unwired: 10 in, 2 out]
            }
          }
        }
        n2094 = call <vilib>:"Add State(s) to Queue__jki_lib_state_machine.vi"("State(s) in (\"\")"=w4723) -> ("States Out"=w4722:string)  [unwired: 14 in]
      }
    }
  }
  n2095 = while {
    shift-right: [w4753] -> _
    shift-left: _ -> [w4752]
    shift-right: [w4756] -> w16
    shift-left: w18 -> [w4750]
    shift-right: [w4755] -> _
    shift-left: w53 -> [w4757]
    tunnel: w7 -> [w4749]
    tunnel: w6 -> [w4748]
    tunnel: w5 -> [w4747]
    tunnel: w4 -> [w4746]
    tunnel: w3 -> [w4745]
    tunnel: [w4744] -> w17
    tunnel: [w4743] -> w14
    tunnel: [w4742] -> w12
    tunnel: [w4741] -> w10
    tunnel: [w4740] -> w8
    i -> [w4739]
    stop <- w4754 stop-if-true
    w4751 = -1  # Timeout
    # "UI State Machine"
    n2096 = call <vilib>:"Parse State Queue__jki_lib_state_machine.vi"("State Queue"=w4757, "Error In (no error)"=w4750) -> ("Remaining States"=w4759:string, "Current State"=w4760:string, "Arguments"=w4758:string)  [unwired: 11 in]
    n2097 = case shown="\"\", \"Idle\"" w4760 {
      selector: w4760 -> [_ _ w4973 _ _ _ _ _]
      tunnel: w4759 -> [w4777 w4967 w4977 w4994 w5004 w5013 w5024 w5037]
      tunnel: w4758 -> [_ _ _ _ _ _ _ _]
      tunnel: w4752 -> [w4775 w4964 w4975 w4991 w5002 w5010 _ w5034]
      tunnel: [w4774 w4965 w4979 errorcluster {"status"=FALSE, "code"=0, "source"=""} ("error out") w5001 w5011 w5021 w5035] -> w4756
      tunnel: w4750 -> [w4773 w4965 w4978 w4990 w5001 w5011 w5021 w5035]
      tunnel: [w4776 w4966 w4976 w4993 w5003 w5012 w5023 w5036] -> w4755
      tunnel: [_ _ _ _ TRUE _ _ _] -> w4754
      tunnel: [w4772 w4964 w4975 w4991 w5002 w5010 w5022 w5034] -> w4753
      tunnel: w4751 -> [w4771 _ _ _ _ _ _ _]
      tunnel: w4749 -> [w4770 w4963 w4972 w4988 w4999 w5009 w5018 w5033]
      tunnel: w4748 -> [w4769 w4962 w4971 w4987 w4998 w5008 w5017 w5032]
      tunnel: w4747 -> [w4768 w4961 w4970 w4986 w4997 w5007 w5016 w5031]
      tunnel: w4746 -> [w4767 w4960 w4969 w4985 w4996 w5006 w5015 w5030]
      tunnel: w4745 -> [w4766 w4959 w4968 w4984 w4995 w5005 w5014 w5029]
      tunnel: [w4765 w4963 w4972 w4988 w4999 w5009 w5018 w5033] -> w4744
      tunnel: [w4764 w4962 w4971 w4987 w4998 w5008 w5017 w5032] -> w4743
      tunnel: [w4763 w4961 w4970 w4986 w4997 w5007 w5016 w5031] -> w4742
      tunnel: [w4762 w4960 w4969 w4985 w4996 w5006 w5015 w5030] -> w4741
      tunnel: [w4761 w4959 w4968 w4984 w4995 w5005 w5014 w5029] -> w4740
      frame "", "Idle" {
        n2098 = event shown="[2] \"GUI Aisle 4.\": Value Change" {
          selector: _ -> [_ _ _ _ _ _ _ _]
          dyn-events: _ -> [_ _ _ _ _ _ _ _]
          timeout: w4771 -> [_ _ _ _ _ _ _ _]
          tunnel: w4777 -> [w4787 w4796 w4818 w4848 w4878 w4908 w4938 w4958]
          tunnel: [w4786 w4795 w4817 w4849 w4879 w4909 w4939 w4957] -> w4776
          tunnel: w4775 -> [w4784 w4794 w4819 w4847 w4877 w4907 w4937 w4955]
          tunnel: [w4785 w4793 w4812 w4841 w4871 w4898 w4933 w4956] -> w4774
          tunnel: w4773 -> [w4785 w4793 w4804 w4837 w4864 w4899 w4926 w4956]
          tunnel: [w4784 w4794 w4819 w4847 w4877 w4907 w4937 w4955] -> w4772
          tunnel: w4770 -> [w4782 w4792 w4810 w4840 w4870 w4893 w4930 w4952]
          tunnel: w4769 -> [w4781 w4791 w4809 w4839 w4869 w4892 w4928 w4951]
          tunnel: w4768 -> [w4780 w4790 w4808 w4838 w4868 w4890 w4920 w4950]
          tunnel: w4767 -> [w4779 w4789 w4800 w4830 w4859 w4889 w4919 w4949]
          tunnel: w4766 -> [w4778 w4788 w4799 w4828 w4858 w4888 w4918 w4948]
          tunnel: [w4782 w4792 w4810 w4840 w4870 w4893 w4929 w4952] -> w4765
          tunnel: [w4781 w4791 w4809 w4839 w4869 w4891 w4928 w4951] -> w4764
          tunnel: [w4780 w4790 w4808 w4838 w4867 w4890 w4920 w4950] -> w4763
          tunnel: [w4779 w4789 w4800 w4829 w4859 w4889 w4919 w4949] -> w4762
          tunnel: [w4778 w4788 w4798 w4828 w4858 w4888 w4918 w4948] -> w4761
          event Timeout {
            n2099 = event-data() -> ()  [unwired: 1 in, 1 out]
            n2100 = call <vilib>:"Add State(s) to Queue__jki_lib_state_machine.vi"("State(s) in Front (\"\")"="" ("State(s) in Front (\"\")"), "State(s) in (\"\")"=w4787) -> ("States Out"=w4786:string)  [unwired: 13 in]
          }
          event "ExitProg": Value Change {
            n2101 = event-data() -> ()  [unwired: 1 in, 6 out]
            n2102 = call <vilib>:"Add State(s) to Queue__jki_lib_state_machine.vi"("State(s) in Front (\"\")"="Exit" ("State(s) in Front (\"\")"), "State(s) in (\"\")"=w4796) -> ("States Out"=w4795:string)  [unwired: 13 in]
          }
          event "GUI Aisle 4.": Value Change {
            n2103 = event-data() -> ()  [unwired: 1 in, 6 out]
            n2104 = local read "File Locations"() -> (w4806:T17[])
            n2105 = local read "GUI Aisle 4."() -> (w4805:T3[])
            n2106 = call "WILT Update Panel.vi"("error in (no error)"=w4804, "GUI Aisle 1A (SLAT)."=w4805, "Location Index"=44 ("x"), "File Locations"=w4806) -> ("error out"=w4803:errorcluster, "Station Data Out"=w4801:T3, "Button Location"=w4802:i32)  [unwired: 5 in]
            n2107 = local read "4"() -> (w4811:T1)
            n2108 = call <vilib>:"Acquire Semaphore.vi"("error in (no error)"=w4803, "semaphore"=w4811) -> ("error out"=w4815:errorcluster, "semaphore out"=w4814:T1)  [unwired: 3 in, 1 out]
            n2109 = flat-sequence {
              tunnel: w4815 -> [w4821]
              tunnel: [w4820] -> w4816
              tunnel: w4814 -> [w4827]
              tunnel: [w4827] -> w4813
              tunnel: w4801 -> [w4826]
              tunnel: w4802 -> [w4825]
              tunnel: w4799 -> [w4823]
              tunnel: [w4822] -> w4798
              frame #0 {
                n2110 = Generate User Event(user event=w4823, event data cluster=TRUE ("Aisle 4"), error in=w4821) -> (user event out=w4822:refnum<user-event>, error out=w4820:errorcluster)  [unwired: 1 in]
                "Aisle 4 Update" <- w4826
                "Aisle 4 Location" <- w4825
              }
            }
            n2111 = call <vilib>:"Release Semaphore.vi"("error in (no error)"=w4816, "semaphore"=w4813) -> ("error out"=w4812:errorcluster)  [unwired: 4 in, 1 out]
            n2112 = call <vilib>:"Add State(s) to Queue__jki_lib_state_machine.vi"("State(s) in (\"\")"=w4818) -> ("States Out"=w4817:string)  [unwired: 14 in]
          }
          event "GUI Aisle 3.": Value Change {
            n2113 = event-data() -> ()  [unwired: 1 in, 6 out]
            n2114 = local read "GUI Aisle 3."() -> (w4835:T3[])
            n2115 = local read "File Locations"() -> (w4833:T17[])
            n2116 = call "WILT Update Panel.vi"("error in (no error)"=w4837, "GUI Aisle 1A (SLAT)."=w4835, "Location Index"=32 ("x"), "File Locations"=w4833) -> ("error out"=w4836:errorcluster, "Station Data Out"=w4831:T3, "Button Location"=w4832:i32)  [unwired: 5 in]
            n2117 = local read "3"() -> (w4842:T1)
            n2118 = call <vilib>:"Acquire Semaphore.vi"("error in (no error)"=w4836, "semaphore"=w4842) -> ("error out"=w4845:errorcluster, "semaphore out"=w4844:T1)  [unwired: 3 in, 1 out]
            n2119 = flat-sequence {
              tunnel: w4845 -> [w4852]
              tunnel: [w4851] -> w4846
              tunnel: w4844 -> [w4857]
              tunnel: [w4857] -> w4843
              tunnel: w4831 -> [w4856]
              tunnel: w4832 -> [w4855]
              tunnel: w4830 -> [w4853]
              tunnel: [w4850] -> w4829
              frame #0 {
                n2120 = Generate User Event(user event=w4853, event data cluster=TRUE ("Aisle 1"), error in=w4852) -> (user event out=w4850:refnum<user-event>, error out=w4851:errorcluster)  [unwired: 1 in]
                "Aisle 3 Update" <- w4856
                "Aisle 3 Location" <- w4855
              }
            }
            n2121 = call <vilib>:"Release Semaphore.vi"("error in (no error)"=w4846, "semaphore"=w4843) -> ("error out"=w4841:errorcluster)  [unwired: 4 in, 1 out]
            n2122 = call <vilib>:"Add State(s) to Queue__jki_lib_state_machine.vi"("State(s) in (\"\")"=w4848) -> ("States Out"=w4849:string)  [unwired: 14 in]
          }
          event "GUI Aisle 2.": Value Change {
            n2123 = event-data() -> ()  [unwired: 1 in, 6 out]
            n2124 = local read "GUI Aisle 2."() -> (w4865:T3[])
            n2125 = local read "File Locations"() -> (w4862:T17[])
            n2126 = call "WILT Update Panel.vi"("error in (no error)"=w4864, "GUI Aisle 1A (SLAT)."=w4865, "Location Index"=20 ("x"), "File Locations"=w4862) -> ("error out"=w4866:errorcluster, "Station Data Out"=w4860:T3, "Button Location"=w4861:i32)  [unwired: 5 in]
            n2127 = local read "2"() -> (w4872:T1)
            n2128 = call <vilib>:"Acquire Semaphore.vi"("error in (no error)"=w4866, "semaphore"=w4872) -> ("error out"=w4875:errorcluster, "semaphore out"=w4874:T1)  [unwired: 3 in, 1 out]
            n2129 = flat-sequence {
              tunnel: w4875 -> [w4883]
              tunnel: [w4882] -> w4876
              tunnel: w4874 -> [w4887]
              tunnel: [w4887] -> w4873
              tunnel: w4860 -> [w4886]
              tunnel: w4861 -> [w4885]
              tunnel: w4868 -> [w4881]
              tunnel: [w4880] -> w4867
              frame #0 {
                n2130 = Generate User Event(user event=w4881, event data cluster=TRUE ("Aisle 1"), error in=w4883) -> (user event out=w4880:refnum<user-event>, error out=w4882:errorcluster)  [unwired: 1 in]
                "Aisle 2 Update" <- w4886
                "Aisle 2 Location" <- w4885
              }
            }
            n2131 = call <vilib>:"Release Semaphore.vi"("error in (no error)"=w4876, "semaphore"=w4873) -> ("error out"=w4871:errorcluster)  [unwired: 4 in, 1 out]
            n2132 = call <vilib>:"Add State(s) to Queue__jki_lib_state_machine.vi"("State(s) in (\"\")"=w4878) -> ("States Out"=w4879:string)  [unwired: 14 in]
          }
          event "GUI Aisle 1A (SLAT).": Value Change {
            n2133 = event-data() -> ()  [unwired: 1 in, 6 out]
            n2134 = local read "GUI Aisle 1A (SLAT)."() -> (w4896:T3[])
            n2135 = local read "File Locations"() -> (w4906:T17[])
            n2136 = call "WILT Update Panel.vi"("error in (no error)"=w4899, "GUI Aisle 1A (SLAT)."=w4896, "Location Index"=12 ("x"), "File Locations"=w4906) -> ("error out"=w4904:errorcluster, "Station Data Out"=w4895:T3, "Button Location"=w4894:i32)  [unwired: 5 in]
            n2137 = local read "1A"() -> (w4900:T1)
            n2138 = call <vilib>:"Acquire Semaphore.vi"("error in (no error)"=w4904, "semaphore"=w4900) -> ("error out"=w4903:errorcluster, "semaphore out"=w4902:T1)  [unwired: 3 in, 1 out]
            n2139 = flat-sequence {
              tunnel: w4903 -> [w4913]
              tunnel: [w4912] -> w4905
              tunnel: w4902 -> [w4917]
              tunnel: [w4917] -> w4901
              tunnel: w4895 -> [w4916]
              tunnel: w4894 -> [w4915]
              tunnel: w4892 -> [w4911]
              tunnel: [w4910] -> w4891
              frame #0 {
                n2140 = Generate User Event(user event=w4911, event data cluster=TRUE ("Aisle 1"), error in=w4913) -> (user event out=w4910:refnum<user-event>, error out=w4912:errorcluster)  [unwired: 1 in]
                "Aisle 1A Update" <- w4916
                "Aisle 1A Location" <- w4915
              }
            }
            n2141 = call <vilib>:"Release Semaphore.vi"("error in (no error)"=w4905, "semaphore"=w4901) -> ("error out"=w4898:errorcluster)  [unwired: 4 in, 1 out]
            n2142 = call <vilib>:"Add State(s) to Queue__jki_lib_state_machine.vi"("State(s) in (\"\")"=w4908) -> ("States Out"=w4909:string)  [unwired: 14 in]
          }
          event "GUI Aisle 1 (SLAT).": Value Change {
            n2143 = event-data() -> ()  [unwired: 1 in, 6 out]
            n2144 = local read "File Locations"() -> (w4925:T17[])
            n2145 = local read "GUI Aisle 1 (SLAT)."() -> (w4923:T3[])
            n2146 = call "WILT Update Panel.vi"("error in (no error)"=w4926, "GUI Aisle 1A (SLAT)."=w4923, "Location Index"=0, "File Locations"=w4925) -> ("error out"=w4927:errorcluster, "Station Data Out"=w4921:T3, "Button Location"=w4922:i32)  [unwired: 5 in]
            n2147 = local read "1"() -> (w4936:T1)
            n2148 = call <vilib>:"Acquire Semaphore.vi"("error in (no error)"=w4927, "semaphore"=w4936) -> ("error out"=w4934:errorcluster, "semaphore out"=w4932:T1)  [unwired: 3 in, 1 out]
            n2149 = flat-sequence {
              tunnel: w4934 -> [w4941]
              tunnel: [w4940] -> w4935
              tunnel: w4932 -> [w4947]
              tunnel: [w4947] -> w4931
              tunnel: w4921 -> [w4946]
              tunnel: w4922 -> [w4945]
              tunnel: w4930 -> [w4943]
              tunnel: [w4942] -> w4929
              frame #0 {
                n2150 = Generate User Event(user event=w4943, event data cluster=TRUE ("Aisle 1"), error in=w4941) -> (user event out=w4942:refnum<user-event>, error out=w4940:errorcluster)  [unwired: 1 in]
                "Aisle 1 Update" <- w4946
                "Aisle 1 Location" <- w4945
              }
            }
            n2151 = call <vilib>:"Release Semaphore.vi"("error in (no error)"=w4935, "semaphore"=w4931) -> ("error out"=w4933:errorcluster)  [unwired: 4 in, 1 out]
            n2152 = call <vilib>:"Add State(s) to Queue__jki_lib_state_machine.vi"("State(s) in (\"\")"=w4938) -> ("States Out"=w4939:string)  [unwired: 14 in]
          }
          event Panel Close? {
            # "Discard the event because we'll close the front panel ourselves in Macro: Exit"
            n2153 = event-data() -> ()  [unwired: 1 in, 1 out]
            n2154 = event-data("Discard?"=TRUE) -> ()  [unwired: 1 in, 1 out]
            n2155 = call <vilib>:"Add State(s) to Queue__jki_lib_state_machine.vi"("State(s) in Front (\"\")"="Exit", "State(s) in (\"\")"=w4958) -> ("States Out"=w4957:string)  [unwired: 13 in]
          }
        }
      }
      frame "---------- Core ----------" {
        # "Do not put any code in this frame.\n(it is a separator no-op)"
        n2156 = call <vilib>:"Add State(s) to Queue__jki_lib_state_machine.vi"("State(s) in (\"\")"=w4967) -> ("States Out"=w4966:string)  [unwired: 14 in]
      }
      frame Default {
        w4982 = 42 items=["No error", "Argument error", "Memory is full", "Out of zone", "End of file", "File already open", "Generic file I/O error", "File not found", "File permission error", "Disk is full", "Duplicate path", "Too many files open", "System feature not enabled", "Resource file not found", "Cannot add resource", "Resource not found", "Image not found", "Image memory error", "Pen does not exist", "Config type invalid", "Config token not found", "Config parse error", "Config memory error", "Bad external code format", "Bad external code offset", "External code not present", "Null window", "Destroy window error", "Null menu", "Print aborted", "Bad print record", "Print driver error", "Windows error during printing", "Memory error during printing", "Print dialog error", "Generic print error", "Invalid device refnum", "Device not found", "Device parameter error", "Device unit error", "Cannot open device", "Device call aborted", "Generic error", "Cancelled by user", "Object ID too low", "Object ID too high", "Object not in heap", "Unknown heap", "Unknown object (invalid DefProc)", "Unknown object (DefProc not in table)", "Message out of range", "Invalid (null) method", "Unknown message", "Manager call not supported", "Bad address", "Network operation in progress", "Network operation timed out", "Connection is busy", "Network attribute not supported", "Network error", "Address in use", "System out of memory", "Connection aborted", "Connection refused", "Not connected", "Already connected", "Connection closed", "Initialization error (interapplication manager)", "Bad occurrence", "Wait on unbound occurrence handler", "Occurrence queue overflow", "Datalog type conflict", "Unused", "Unrecognized type (interapplication manager)", "Memory corrupt", "Failed to make temporary DLL", "Old CIN version", "Drag socket not found", "Failed to load drop-object", "Failed to register OLE object", "Failed to release OLE object", "Format specifier type mismatch", "Unknown format specifier", "Too few format specifiers", "Too many format specifiers", "Scan failed", "Newer CIN version", "Error converting to variant", "Runtime menu error", "Password tampered", "Variant attribute not found", "Incompatible variant data type", "Event data is not available", "Event Store is not present", "Occurrence is not found", "Event Queue is not created", "Event info is not available", "Refnum passed is NULL", "Error retrieving Class GUID", "Error retrieving CoClass GUID", "Error retrieving TypeLib GUID.", "Bad built application magic bytes.", "Specific driver is different from the specific driver associated with the Logical Name.", "There is no session opened to the class driver.", "Max Error", "MAX - Error with config objects", "MAX - Error loading configuration", "MAX - Group not supported"]
        # "Current State"
        # "Do not delete, rename, or modify this frame.\n(this is used to capture unhandled states and typos)"
        # "Handle mistyped state name (developer tool)"
        n2157 = Format Into String(format string="Software Exception: Unhandled State \"%s\"." ("message"), error in=w4978, w4973) -> (resulting string=w4981:string, error out=w4980:errorcluster)  [unwired: 1 in]
        n2158 = call <vilib>:"Error Cluster From Error Code.vi"("show call chain? (False)"=TRUE, "error in (no error)"=w4980, "error message (\"\")"=w4981, "error code (0)"=w4982) -> ("error out"=w4979:errorcluster)  [unwired: 5 in]
        n2159 = call <vilib>:"Add State(s) to Queue__jki_lib_state_machine.vi"("State(s) in (\"\")"=w4977) -> ("States Out"=w4976:string)  [unwired: 14 in]
      }
      frame "Error Handler" {
        # "Unhandled Error -- Display it"
        # "Handle any errors here.\nYou can also output any states to clean-up after errors occur"
        # "Clear error"
        n2160 = call <vilib>:"General Error Handler.vi"("error in (no error)"=w4990) -> ()  [unwired: 10 in, 5 out]
        n2161 = call <vilib>:"Add State(s) to Queue__jki_lib_state_machine.vi"("State(s) in Front (\"\")"="/* Post Error States", "State(s) in (\"\")"=w4994) -> ("States Out"=w4993:string)  [unwired: 13 in]
      }
      frame "Exit" {
        # "Do not put any code in this frame.\n(No errors that occur here will be handled.)"
        n2162 = call <vilib>:"Add State(s) to Queue__jki_lib_state_machine.vi"("State(s) in (\"\")"=w5004) -> ("States Out"=w5003:string)  [unwired: 14 in]
      }
      frame "---------- Data ----------" {
        n2163 = call <vilib>:"Add State(s) to Queue__jki_lib_state_machine.vi"("State(s) in (\"\")"=w5013) -> ("States Out"=w5012:string)  [unwired: 14 in]
      }
      frame "Data: Initialize" {
        n2164 = while {
          tunnel: [w5028] -> w5020
          tunnel: [w5027] -> w5019
          stop <- w5026 stop-if-true
          w5027 = ""  # Your string data
          w5028 = TRUE  # Your Boolean data
          n2165 = local read "Initialization Complete"() -> (w5026:bool)
          n2166 = Wait Until Next ms Multiple(millisecond multiple=u32 100) -> ()  [unwired: 1 out]
        }
        n2167 = Bundle("Your Boolean data"=w5020, "Your string data"=w5019) -> (w5022:T38)  [unwired: 1 in]
        n2168 = call <vilib>:"Add State(s) to Queue__jki_lib_state_machine.vi"("State(s) in (\"\")"=w5024) -> ("States Out"=w5023:string)  [unwired: 14 in]
      }
      frame "---------- Check Status ----------" {
        n2169 = call <vilib>:"Add State(s) to Queue__jki_lib_state_machine.vi"("State(s) in (\"\")"=w5037) -> ("States Out"=w5036:string)  [unwired: 14 in]
      }
    }
    "UI Runs" <- w4739
  }
  n2170 = Destroy User Event(user event=w45, error in=w42) -> ()  [unwired: 1 out]
  n2171 = Destroy User Event(user event=w17, error in=w16) -> (error out=w15:errorcluster)
  n2172 = Release Notifier(notifier=w32, error in (no error)=w31) -> (error out=→"Error Out":errorcluster)  [unwired: 1 in, 2 out]
  n2173 = Destroy User Event(user event=w14, error in=w15) -> (error out=w13:errorcluster)
  n2174 = Destroy User Event(user event=w12, error in=w13) -> (error out=w11:errorcluster)
  n2175 = Destroy User Event(user event=w10, error in=w11) -> (error out=w9:errorcluster)
  n2176 = Destroy User Event(user event=w8, error in=w9) -> ()  [unwired: 1 out]
